vi "Seitenumbruch test.vi"() -> ()   [LabVIEW 2015, in "Linearisierung v2.lvlib" / "Protokoll.lvlib"]
uses:
  Protokoll.lvlib
  <vilib>/Utility/miscctls.llb/LVPrintingMarginsTypeDef.ctl
panel:
  out "XY-Graph EPA 2":cluster{dbl[], dbl[]}[](graph) caption="XY-Graph"
  out "Ergebnis:":string
  out "Konzentration:":string
  out "Komponente:":string
  out "Bearbeiter:":string
  out "Gasteiler:":string
  out "Messgerät:":string
  out "EPA Auswertung":string[][](table) caption="Evaluation"
  out "XY-Graph EPA":cluster{dbl[], dbl[]}[](graph) caption="XY-Graph"
  out "EPA Ausgabetabelle":string[][](table)
  # "Linearity Check EPA §1065.307"
  # "Linearity detection §1065.307"
  # "Description of the limits"
  # "Slope (a1) value between 0,99-1,01"
  # "Intercept (a0)"
  # "laboratory: Value <= 0,5% of the gas concentration"
  # "field: Value <= 1% of the gas concentration"
  # "Coefficient of determination (R²) Value >= 0,998"
  # "standard error of estimate (SEE) Value <= 1% of the gas concentration"
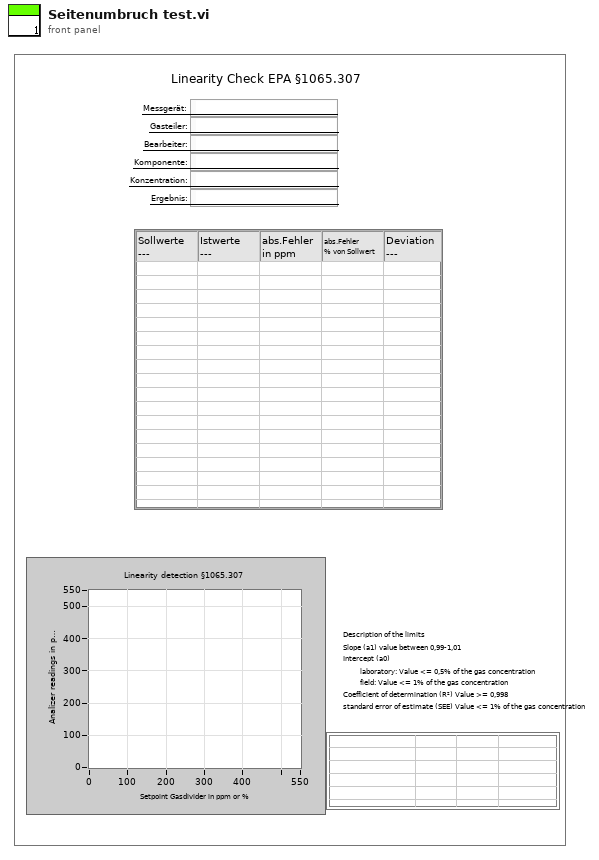
[diagram p1: front panel]
types:
  T1 = enum32{"Portrait", "Landscape", "Rotated Portrait", "Rotated Landscape"}
  T2 = enum32{"Custom", "Standard", "Using Panel", "Using SubVI", "Complete"}
  T3 = typedef "LVPrintingMarginsTypeDef.ctl" = cluster{"Top":sgl, "Left":sgl, "Bottom":sgl, "Right":sgl, "Measurement System":enum8{"Inches", "cm"}}
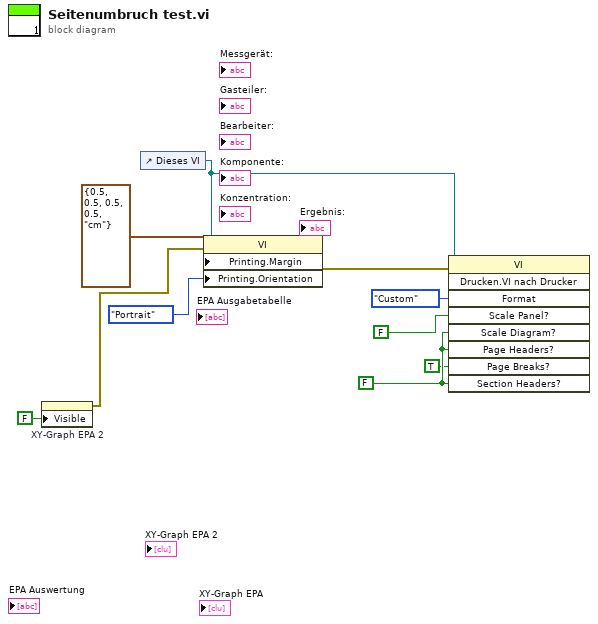
[diagram p0: block diagram]
diagram:
  w4 = FALSE ("Abschnittskopfzeilen?")
  n1 = property on="XY-Graph EPA 2" class="XYGraph (strikt)"("Visible"=FALSE ("Sichtbar")) -> (error out=w1:errorcluster)  [unwired: 2 in, 1 out]
  n2 = control-ref of="Dieses VI"() -> (w10:refnum<vi>)
  n3 = property class="VI"(reference=w10, error in=w1, "Printing.Margin"=T3 {"Top"=0.5, "Left"=0.5, "Bottom"=0.5, "Right"=0.5, "Measurement System"=enum."cm"} ("Drucken:Ränder"), "Printing.Orientation"=T1."Portrait" ("Drucken:Seitenausrichtung")) -> (error out=w8:errorcluster)  [unwired: 1 out]
  n4 = invoke class="VI" method="Drucken.VI nach Drucker"(reference=w10, error in=w8, "Format"=T2."Custom" ("Formatieren"), "Scale Panel?"=FALSE ("Panel skalieren?"), "Scale Diagram?"=w4, "Page Headers?"=w4, "Page Breaks?"=TRUE ("Seitenumbrüche?"), "Section Headers?"=w4) -> ()  [unwired: 1 in, 9 out]
